vi "Init DIO page.vi"(6 "Card Position":refnum<vi>, 7 "IO Settings":refnum<vi>, 8 "error in (no error)":errorcluster, 9 "Description":refnum<vi>, 10 "Name":refnum<vi>, 11 "Node Ptr":T1 format="%.0x") -> (0 "error out":errorcluster, 3 "Node Ptr out":T1=18446744073709551615 format="%.0x")   [LabVIEW 2013, in "SLSC configuration System Explorer.lvlib"]
uses:
  SLSC configuration System Explorer.lvlib
  <vilib>/NI Veristand/Custom Device API/Custom Device Item Ref.ctl
  Shared/Card Postion.ctl
  Shared/DIO card config.ctl
  Shared/Constants.vi
  <vilib>/NI Veristand/Custom Device API/Get Item Property (Variant).vi
  <vilib>/NI Veristand/Custom Device API/Custom Device API.lvlib
  Shared/SLSC configuration Shared.lvlib
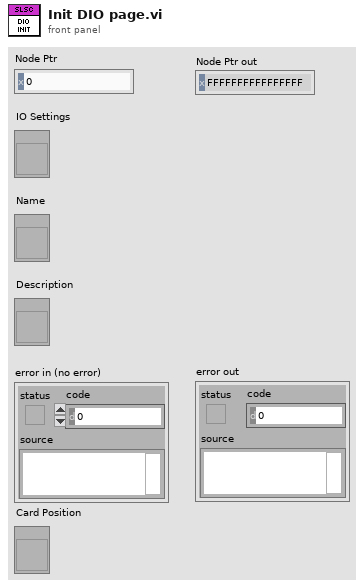
[diagram p1: front panel]
types:
  T1 = typedef "Custom Device API.lvlib/Custom Device Item Ref.ctl" = u64
  T2 = typedef "SLSC configuration Shared.lvlib/Card Postion.ctl" = cluster{"Chassis #":u8, "Slot #":u8}
  T3 = typedef "SLSC configuration Shared.lvlib/DIO card config.ctl" = cluster{"Byte 1":cluster{"Line 1":bool, "Line 2":bool, "Line 3":bool, "Line 4":bool, "Line 5":bool, "Line 6":bool, "Line 7":bool, "Line 8":bool, "Logic Threshold (%)":u32}, "Byte 2":cluster{"Line 1":bool, "Line 2":bool, "Line 3":bool, "Line 4":bool, "Line 5":bool, "Line 6":bool, "Line 7":bool, "Line 8":bool, "Logic Threshold (%)":u32}, "Byte 3":cluster{"Line 1":bool, "Line 2":bool, "Line 3":bool, "Line 4":bool, "Line 5":bool, "Line 6":bool, "Line 7":bool, "Line 8":bool, "Logic Threshold (%)":u32}, "Byte 4":cluster{"Line 1":bool, "Line 2":bool, "Line 3":bool, "Line 4":bool, "Line 5":bool, "Line 6":bool, "Line 7":bool, "Line 8":bool, "Logic Threshold (%)":u32}}
  T4 = typedef "Custom Device API.lvlib/Custom Device Item Info.ctl" = cluster{"Name":string, "Is Channel":bool, "GUID":string, "Is Waveform":bool}
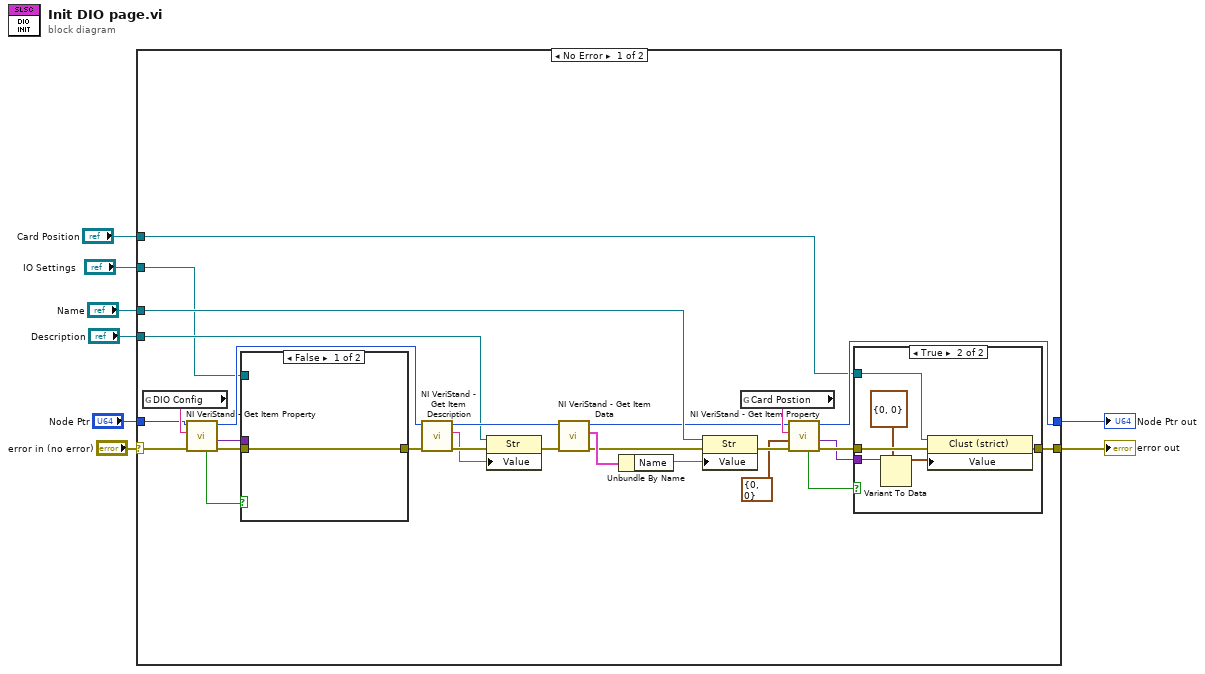
[diagram p0: block diagram]
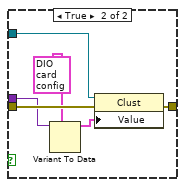
[diagram p3: hidden frame]
diagram:
  n1 = case shown="No Error" "error in (no error)" {
    selector: "error in (no error)" -> [w35 w52]
    tunnel: "Node Ptr" -> [w32 w51]
    tunnel: [w15 w51] -> w3
    tunnel: [w17 w52] -> w4
    tunnel: "Description" -> [w23 _]
    tunnel: "Name" -> [w22 _]
    tunnel: "IO Settings" -> [w21 _]
    tunnel: "Card Position" -> [w13 _]
    frame No Error {
      n2 = global read "Constants.vi" "DIO Config"() -> (w36:string)
      n3 = call-poly <vilib>:"NI VeriStand - Get Item Property.vi"("error in (no error)"=w35, "Property Name"=w36, "Item Ref in"=w32) -> ("error out"=w34:errorcluster, "Value"=w11:variant, "Item Ref out"=w31:T1, "Found?"=w10:bool)  [unwired: 5 in]
      n4 = case shown="False" w10 {
        tunnel: w34 -> [w44 w50]
        tunnel: [w44 w49] -> w33
        tunnel: w21 -> [_ w45]
        tunnel: w11 -> [_ w48]
        frame False {
        }
        frame True {
          n5 = Variant To Data(type=T3 {"Byte 1"={"Line 1"=FALSE, "Line 2"=FALSE, "Line 3"=FALSE, "Line 4"=FALSE, "Line 5"=FALSE, "Line 6"=FALSE, "Line 7"=FALSE, "Line 8"=FALSE, "Logic Threshold (%)"=0}, "Byte 2"={"Line 1"=FALSE, "Line 2"=FALSE, "Line 3"=FALSE, "Line 4"=FALSE, "Line 5"=FALSE, "Line 6"=FALSE, "Line 7"=FALSE, "Line 8"=FALSE, "Logic Threshold (%)"=0}, "Byte 3"={"Line 1"=FALSE, "Line 2"=FALSE, "Line 3"=FALSE, "Line 4"=FALSE, "Line 5"=FALSE, "Line 6"=FALSE, "Line 7"=FALSE, "Line 8"=FALSE, "Logic Threshold (%)"=0}, "Byte 4"={"Line 1"=FALSE, "Line 2"=FALSE, "Line 3"=FALSE, "Line 4"=FALSE, "Line 5"=FALSE, "Line 6"=FALSE, "Line 7"=FALSE, "Line 8"=FALSE, "Logic Threshold (%)"=0}} ("Cluster"), Variant=w48) -> (data=w47:T3)  [unwired: 1 in, 1 out]
          n6 = property class="Clust"(reference=w45, error in=w50, "Value"=w47) -> (error out=w49:errorcluster)  [unwired: 1 out]
        }
      }
      n7 = call <vilib>:"NI VeriStand - Get Item Description.vi"("error in (no error)"=w33, "Item Ref in"=w31) -> ("error out"=w30:errorcluster, "Description"=w29:string, "Item Ref out"=w24:T1)  [unwired: 7 out]
      n8 = property class="Str"(reference=w23, error in=w30, "Value"=w29) -> (error out=w27:errorcluster)  [unwired: 1 out]
      n9 = call <vilib>:"NI VeriStand - Get Item Data.vi"("error in (no error)"=w27, "Item Ref in"=w24) -> ("error out"=w26:errorcluster, "Item Info"=w28:T4, "Item Ref out"=w16:T1)  [unwired: 7 out]
      n10 = Unbundle By Name(w28) -> ("Name"=w25:string)
      n11 = property class="Str"(reference=w22, error in=w26, "Value"=w25) -> (error out=w18:errorcluster)  [unwired: 1 out]
      n12 = global read "Constants.vi" "Card Postion"() -> (w19:string)
      n13 = call-poly <vilib>:"NI VeriStand - Get Item Property.vi"("error in (no error)"=w18, "Default Value"=T2 {"Chassis #"=0, "Slot #"=0} ("Card Position"), "Property Name"=w19, "Item Ref in"=w16) -> ("error out"=w20:errorcluster, "Value"=w14:variant, "Item Ref out"=w15:T1, "Found?"=w9:bool)  [unwired: 4 in]
      n14 = case shown="True" w9 {
        tunnel: w20 -> [w37 w43]
        tunnel: [w37 w42] -> w17
        tunnel: w14 -> [_ w41]
        tunnel: w13 -> [_ w38]
        frame False {
        }
        frame True {
          n15 = Variant To Data(type=T2 {"Chassis #"=0, "Slot #"=0} ("Card Position"), Variant=w41) -> (data=w40:T2)  [unwired: 1 in, 1 out]
          n16 = property class="Clust (strict)"(reference=w38, error in=w43, "Value"=w40) -> (error out=w42:errorcluster)  [unwired: 1 out]
        }
      }
    }
    frame Error {
    }
  }
  "error out" <- w4
  "Node Ptr out" <- w3
